vi "HatchLineupvi.vi"() -> ()   [LabVIEW 2018]
uses:
  <vilib>/Rock Robotics/WPI/Solenoid/WPI_SolenoidValue.ctl
  <vilib>/addons/control/pid/pid.llb/PID (DBL).vi
  <vilib>/Rock Robotics/WPI/Solenoid/WPI_SolenoidSetEnum.vi
  <vilib>/addons/control/pid/NI_PID_pid.lvlib
panel:
  out "Strafe Motor":dbl format="%#_13g"
  in  "Move Forward Power":dbl format="%#_13g"
  in  "Move Forward Max/Min":cluster{"output high":dbl, "output low":dbl}={"output high"=100.0, "output low"=-100.0} {"output low" format="%.2f"; "output high" format="%.2f"}
  in  "Move Forward PID Values":T1={"proportional gain (Kc)"=1.0, "integral time (Ti, min)"=0.01, "derivative time (Td, min)"=0.0}
  in  "Pos PID Values":T1={"proportional gain (Kc)"=1.0, "integral time (Ti, min)"=0.01, "derivative time (Td, min)"=0.0}
  out "Right Motor":dbl format="%#_13g"
  out "Left Motor":dbl format="%#_13g"
  in  "Pos Max/Min":cluster{"output high":dbl, "output low":dbl}={"output high"=100.0, "output low"=-100.0} {"output low" format="%.2f"; "output high" format="%.2f"}
  in  "Pos":dbl format="%#_13g"
  in  "Rot":dbl format="%#_13g"
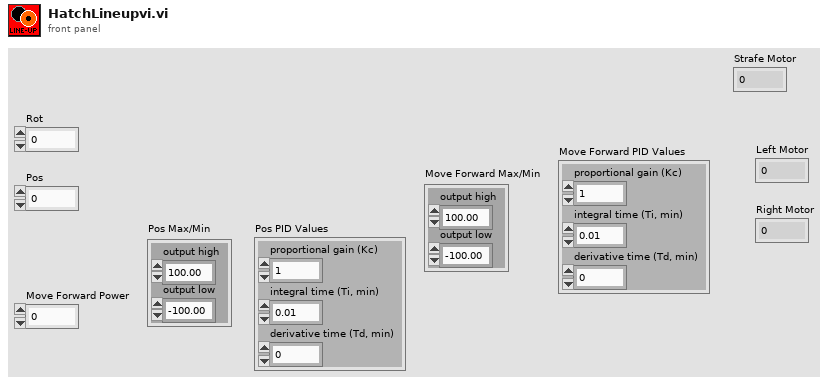
[diagram p1: front panel]
types:
  T1 = cluster{"proportional gain (Kc)":dbl, "integral time (Ti, min)":dbl, "derivative time (Td, min)":dbl}
  T2 = typedef "WPI_SolenoidDevRef.ctl" = cluster{"DevStatus":errorcluster, "Pneumatics Control Module":u8, "Forward Solenoid Channel":T3, "Reverse Solenoid Channel":T3}
  T3 = typedef "WPI_SolenoidChannel.ctl" = enum8{"Solenoid 0", "Solenoid 1", "Solenoid 2", "Solenoid 3", "Solenoid 4", "Solenoid 5", "Solenoid 6", "Solenoid 7", "Invalid"}
  T4 = typedef "WPI_SolenoidValue.ctl" = enum16{"Off", "On", "Forward", "Reverse"}
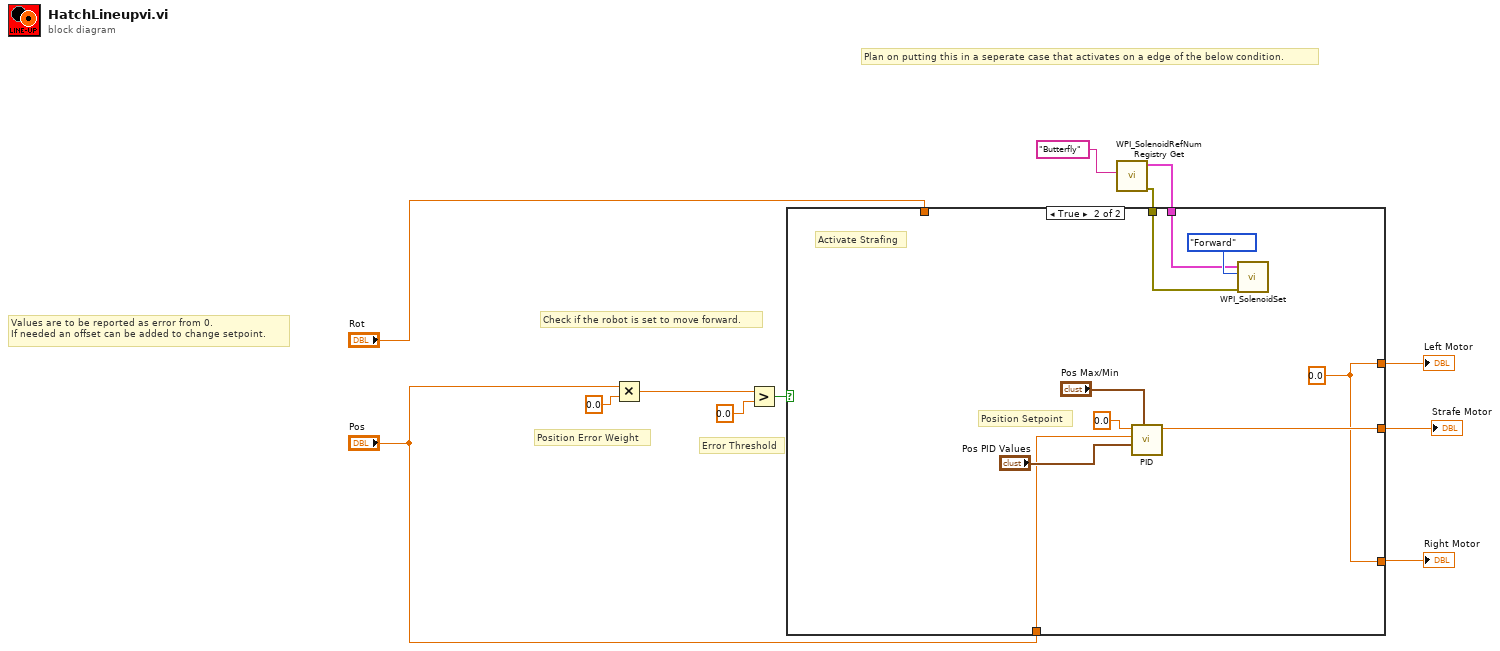
[diagram p0: block diagram]
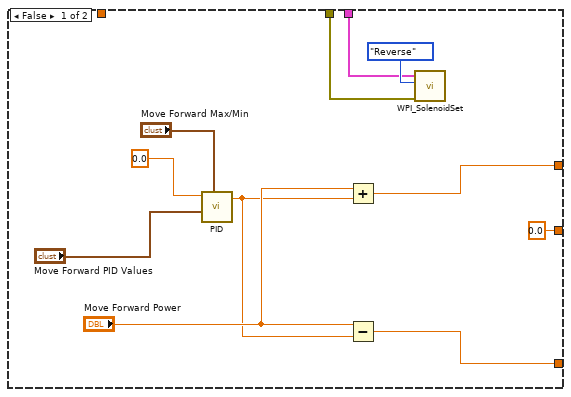
[diagram p2: hidden frame]
diagram:
  # "Values are to be reported as error from 0. \nIf needed an offset can be added to change setpoint."
  # "Plan on putting this in a seperate case that activates on a edge of the below condition."
  # "Error Threshold"
  # "Position Error Weight"
  # "Check if the robot is set to move forward."
  n1 = Multiply(x="Pos", y=0.0) -> (x*y=w1:dbl)
  n2 = Greater?(x=w1, y=0.0) -> (0:w12:bool)
  n3 = call <vilib>:"WPI_SolenoidRefNum Registry Get.vi"("refnum name"="Butterfly") -> ("error out"=w4:errorcluster, "SolenoidDevRef"=w3:T2)  [unwired: 9 in]
  n4 = case shown="True" w12 {
    tunnel: "Rot" -> [_ _]
    tunnel: "Pos" -> [_ w29]
    tunnel: [w17 w24] -> w7
    tunnel: [w18 w24] -> w6
    tunnel: w4 -> [w15 w27]
    tunnel: w3 -> [w14 w26]
    tunnel: [0.0 ("output") w25] -> w2
    frame False {
      n5 = call-poly <vilib>:"PID.vi"("output range"="Move Forward Max/Min", "PID gains"="Move Forward PID Values", "setpoint"=0.0) -> ("output"=w19:dbl)  [unwired: 7 in, 1 out]
      n6 = Add(x="Move Forward Power", y=w19) -> (x+y=w18:dbl)
      n7 = Subtract(x="Move Forward Power", y=w19) -> (x-y=w17:dbl)
      n8 = call-poly <vilib>:"WPI_SolenoidSet.vi"("error in (no error)"=w15, "Value"=WPI_SolenoidValue."Reverse", "SolenoidDevRef"=w14) -> ()  [unwired: 7 in, 2 out]
    }
    frame True {
      w24 = 0.0
      # "Position Setpoint"
      # "Activate Strafing"
      n9 = call-poly <vilib>:"PID.vi"("output range"="Pos Max/Min", "PID gains"="Pos PID Values", "process variable"=w29, "setpoint"=0.0) -> ("output"=w25:dbl)  [unwired: 6 in, 1 out]
      n10 = call-poly <vilib>:"WPI_SolenoidSet.vi"("error in (no error)"=w27, "Value"=WPI_SolenoidValue."Forward", "SolenoidDevRef"=w26) -> ()  [unwired: 7 in, 2 out]
    }
  }
  "Left Motor" <- w6
  "Right Motor" <- w7
  "Strafe Motor" <- w2
